vi "Main Tclk.vi"() -> ()   [LabVIEW 2018] (continued)
      n182 = local write "Beam dump at zero"(w117) -> ()
      n183 = local write "EHT off"(w117) -> ()
      n184 = local write "Temperature warning armed"(w117) -> ()
      n185 = local write "Auto Align"(w117) -> ()
      n186 = local write "Auto re-engage"(w117) -> ()
      n187 = local write "Off"(w117) -> ()
      n188 = local write "Spot"(w117) -> ()
      n189 = local write "Auto Stig"(w117) -> ()
      n190 = local write "FIB Profile"(w117) -> ()
      n191 = shared-variable "My Computer\\Zeiss Library.lvlib\\Milling Line Paused"(w117) -> ()  [unwired: 1 in, 1 out]
      n192 = local write "dat to csv and xml"(w117) -> ()
      n193 = local write "Send reheat start email"(w117) -> ()
      n194 = local write "Mouse down"(w117) -> ()
      n195 = call-poly <vilib>:"DAQmx Create Virtual Channel.vi"("physical channels"=w274) -> ("task out"=w272:refnum<k21>, "error out"=w273:errorcluster)  [unwired: 13 in]
      n196 = local write "Mill Stop"(w117) -> ()
      n197 = local write "Stop"(w117) -> ()
      n198 = local write "ROI"(w117) -> ()
      n199 = property on="Reheat Parameters" class="Clust (strict)"("Visible"=w175) -> ()  [unwired: 2 in, 2 out]
      n200 = property on="FIB Parameters" class="Clust (strict)"("Visible"=w177) -> ()  [unwired: 2 in, 2 out]
      n201 = property on="HV Data Output" class="Clust (strict)"("Visible"=w176) -> ()  [unwired: 2 in, 2 out]
      n202 = property on="Capella HV Data Output" class="Clust (strict)"("Visible"=w114) -> ()  [unwired: 2 in, 2 out]
      n203 = Unbundle By Name(w273) -> ("status"=w271:bool)
      n204 = local write "Auto Focus"(w117) -> ()
      n205 = shared-variable "My Computer\\Zeiss Library.lvlib\\Stop"(w117) -> ()  [unwired: 1 in, 1 out]
      n206 = local write "Scan x1"(w117) -> ()
      n207 = local write "FIB time lapse"(w117) -> ()
      n208 = local write "Reheat from last"(w117) -> ()
      n209 = local write "SEM Status"(w326) -> ()
      n210 = local read "FIB Scan Parameters"() -> (w317:T32)
      n211 = expression code="x/2"(w278) -> (w279:dbl)
      n212 = local write "Request to reheat"(w117) -> ()
      n213 = local write "Mill"(w117) -> ()
      n214 = case shown="False" w271 {
        tunnel: w272 -> [w600 _]
        frame False {
          n215 = call <vilib>:"DAQmx Clear Task.vi"("task in"=w600) -> ()  [unwired: 14 in, 1 out]
          n216 = property on="Sweep enabled" class="Bool (strict)"("DisabledEnum"=T44."Enabled" ("Disabled")) -> ()  [unwired: 2 in, 2 out]
        }
        frame True {
          n217 = local write "Sweep enabled"(FALSE ("Sweep enabled")) -> ()
          n218 = property on="Sweep enabled" class="Bool (strict)"("DisabledEnum"=T44."Disabled and Grayed Out" ("Disabled")) -> ()  [unwired: 2 in, 2 out]
        }
      }
      n219 = local write "Re-engage cancelled"(w117) -> ()
      n220 = property on="COM port" class="VISAName"("DisabledEnum"=w277) -> ()  [unwired: 2 in, 2 out]
      n221 = local write "Focus index stop trigger active"(w117) -> ()
      n222 = local read "Milling para"() -> (w313:T35)
      n223 = Bundle By Name(cluster=w313, "FIB FOV (um)"=w278, "Mill from Bottom"=FALSE, "X size (um)"=w279, "Z size (um)"=w279) -> (w312:T35)
      n224 = local read "Alert Settings"() -> (w233:T36)
      n225 = Bundle By Name(cluster=w233, "Low limit"=w232, "High limit"=w231) -> (w230:T36)
      n226 = local read "SEM Options"() -> (w306:T27)
      n227 = property on="Start FIB HV DataLog" class="Bool (strict)"("Visible"=w206) -> ()  [unwired: 2 in, 2 out]
      n228 = property on="Low limit" class="DigNum (strict)"("Caption.Text"=w242) -> ()  [unwired: 2 in, 2 out]
      n229 = property on="High limit" class="DigNum (strict)"("Caption.Text"=w241) -> ()  [unwired: 2 in, 2 out]
      n230 = property on="Faraday Cup (nA)" class="DigNum (strict)"("Caption.Text"=w239) -> ()  [unwired: 2 in, 2 out]
      n231 = property on="Faraday Cup log" class="XYGraph (strict)"("YScale.NameLbl.Text"=w238) -> ()  [unwired: 2 in, 2 out]
      n232 = property on="Config Tabs" class="TabCtl (strict)"() -> ("Pages"=w211:refnum<vi>[])  [unwired: 2 in, 2 out]
      n233 = local write "FIB"(w117) -> ()
      n234 = Bundle By Name(cluster=w317, "X size (V)"=w315, "Z size (V)"=w315) -> (w316:T32)
      n235 = local write "Mill Manual Pause"(w117) -> ()
      n236 = local write "FIB-SEM Angle"(w314) -> ()
      n237 = local read "FIB Options"() -> (w310:T33)
      n238 = property on="SEM HV Data Output" class="Clust (strict)"("Visible"=w114) -> ()  [unwired: 2 in, 2 out]
      n239 = local write "3D FIB-SEM"(w117) -> ()
      n240 = local write "Pause for reheat"(w117) -> ()
      n241 = local write "Request to stop reheat"(w117) -> ()
      n242 = property on="Extractor (kV)" class="DigNum (strict)"("Visible"=w199) -> ()  [unwired: 2 in, 2 out]
      n243 = Bundle By Name(cluster=w310, "Flip x"=w168, "Flip z"=TRUE ("data")) -> (w309:T33)
      n244 = Index Array(array=w211, index=T43."FIB Reheat" ("Config Tabs")) -> (element=w210:refnum<vi>)
      n245 = local write "Alert Settings"(w230) -> ()
      n246 = Bundle By Name(cluster=w306, "Detector A"=w304, "Detector B"=w303) -> (w305:T27)
      n247 = local read "Milling para"() -> (w324:T35)
      n248 = Bundle By Name(cluster=w324, "Auto pause"=w258, "Mill start from Last"=w258) -> (w323:T35)
      n249 = local write "Start Current DataLog"(w117) -> ()
      n250 = xnode "Match Regular Expression"("input string"=w182, "regular expression"="Merlin", "ignore case? (F)"=TRUE) -> ("offset past match"=w269:i32)  [unwired: 3 in, 4 out]
      n251 = xnode "Match Regular Expression"("input string"=w182, "regular expression"="Gemini500", "ignore case? (F)"=TRUE) -> ("offset past match"=w184:i32)  [unwired: 3 in, 4 out]
      n252 = property class="Page"(reference=w210, "PageEnb"=w144) -> ()  [unwired: 1 in, 2 out]
      n253 = local write "FIB Imaging"(w117) -> ()
      n254 = property on="Turn FIB gun standby" class="Bool (strict)"("Visible"=w114) -> ()  [unwired: 2 in, 2 out]
      n255 = local write "FIB Options"(w309) -> ()
      n256 = Equal?(x=w269, y=-1) -> (x = y?=w181:bool)
      n257 = Equal?(x=w184, y=-1) -> (x = y?=w180:bool)
      n258 = local write "FIB Scan Parameters"(w316) -> ()
      n259 = local write "Cancel Auto re-engage"(w117) -> ()
      n260 = property on="13nA Condenser (V)" class="DigNum (strict)"("Visible"=w199) -> ()  [unwired: 2 in, 2 out]
      n261 = local write "Milling para"(w312) -> ()
      n262 = local write "Status message"("standby" ("Status message")) -> ()
      n263 = local write "SEM Options"(w305) -> ()
      n264 = And(x=w181, y=w180) -> (x .and. y?=w179:bool)
      n265 = local write "Reheat completed"(w117) -> ()
      n266 = property on="Status Tabs" class="TabCtl (strict)"() -> ("Pages"=w207:refnum<vi>[])  [unwired: 2 in, 2 out]
      n267 = local write "Unfreeze"(w117) -> ()
      n268 = local write "Scan xn"(w117) -> ()
      n269 = Square Root(x=sgl 2.0 ("t")) -> (sqrt(x)=w118:sgl)
      n270 = local write "Milling para"(w323) -> ()
      n271 = property on="27nA Condenser (V)" class="DigNum (strict)"("Visible"=w199) -> ()  [unwired: 2 in, 2 out]
      n272 = property on="Reheat Output" class="Clust (strict)"("Visible"=w206) -> ()  [unwired: 2 in, 2 out]
      n273 = property on="Turn off FIB gun" class="Bool (strict)"("Visible"=w114) -> ()  [unwired: 2 in, 2 out]
      n274 = property on="Suppressor (V)" class="DigNum (strict)"("Visible"=TRUE) -> ()  [unwired: 2 in, 2 out]
      n275 = Divide(x=w119, y=w118) -> (x/y=w120:sgl)
      n276 = Index Array(array=w207, index=T11."HV Data" ("Status Tabs")) -> (element=w208:refnum<vi>)
      n277 = Select(t=w119, s=w179, f=w120) -> (s? t:f=w178:sgl)
      "X full scale (V)" <- w178
      n278 = property class="DAQmx Device"("Active Device"=w266) -> (error out=w260:errorcluster, "AI.PhysicalChans"=w265:tag[])  [unwired: 2 in, 1 out]
      "Logging Channels" <- w265
      n279 = local read "File Information"() -> (w308:T31)
      n280 = property class="Page"(reference=w208, "PageEnb"=w144) -> ()  [unwired: 1 in, 2 out]
      n281 = shared-variable ".\\Zeiss Library.lvlib\\X full scale (V)"(w178) -> ()  [unwired: 1 in, 1 out]
      n282 = property on="Open FIB gun valve" class="Bool (strict)"("Visible"=w114) -> ()  [unwired: 2 in, 2 out]
      n283 = property on="Image Tabs" class="TabCtl (strict)"() -> ("Pages"=w146:refnum<vi>[])  [unwired: 2 in, 2 out]
      n284 = Unbundle By Name(w260) -> ("status"=w259:bool)
      n285 = Bundle By Name(cluster=w308, "File path"=path "E:/Images", "Save recipe"=w125, "Load recipe"=w125) -> (w307:T31)
      n286 = property on="Cursor Z (V)" class="DigNum (strict)"("Visible"=w125) -> ()  [unwired: 2 in, 2 out]
      n287 = Array Size(array="Parameter Names") -> (size(s)=w262:i32)
      n288 = shared-variable ".\\Zeiss Library.lvlib\\Upload flags path"("D:\\UploadFlags" ("string")) -> ()  [unwired: 1 in, 1 out]
      n289 = property on="FIB Gun Valve Status" class="Str"("Visible"=w114) -> ()  [unwired: 2 in, 2 out]
      n290 = Index Array(array=w146, index=T37."FIB HV Data" ("Image Tabs")) -> (element=w145:refnum<vi>)
      n291 = Array Subset(array=w265, length=w262) -> (w264:tag[])  [unwired: 1 in]
      n292 = Build Path(base path=w129, name or relative path="Email Log") -> (appended path=w215:path)
      "Email Log Files" <- w215
      n293 = Build Path(base path=w129, name or relative path="FIB HV DataLog") -> (appended path=w219:path)
      "FIB HV DataLog Files" <- w219
      n294 = Build Path(base path=w129, name or relative path="SEM HV DataLog") -> (appended path=w169:path)
      "SEM HV DataLog Files" <- w169
      n295 = Build Path(base path=w129, name or relative path="Current DataLog") -> (appended path=w166:path)
      "Current DataLog Files" <- w166
      n296 = Build Path(base path=w129, name or relative path="FIB Reheat Log") -> (appended path=w197:path)
      "FIB Reheat Log Files" <- w197
      n297 = Build Path(base path=w129, name or relative path="Re-engage") -> (appended path=w131:path)
      "Re-engage Files" <- w131
      n298 = Build Path(base path=w129, name or relative path="FIB Probes.csv") -> (appended path=w132:path)
      n299 = Build Path(base path=w129, name or relative path="Last FIB milling snapshot.xml") -> (appended path=→"Last milling snapshot":path)
      n300 = Build Path(base path=w129, name or relative path="Last FIB recipe.csv") -> (appended path=→"Last FIB recipe":path)
      n301 = Build Path(base path=w129, name or relative path="Last FIB image.png") -> (appended path=→"Last FIB image":path)
      n302 = Build Path(base path=w129, name or relative path="Last FIB zoom pre image.png") -> (appended path=→"Last FIB zoom pre image":path)
      n303 = Build Path(base path=w129, name or relative path="Last DetA LM image.png") -> (appended path=→"Last Det A Low Mag":path)
      n304 = Build Path(base path=w129, name or relative path="Last DetB LM image.png") -> (appended path=→"Last Det B Low Mag":path)
      n305 = Build Path(base path=w129, name or relative path="Email alert recipients.txt") -> (appended path=w226:path)
      "Email recipents file" <- w226
      n306 = property class="Page"(reference=w145, "PageEnb"=w144) -> ()  [unwired: 1 in, 2 out]
      n307 = property on="FIB Milling Objective (V)" class="DigNum (strict)"("Visible"=w114) -> ()  [unwired: 2 in, 2 out]
      n308 = property on="FIB Milling Probe" class="CmbBox"("Visible"=w114) -> ()  [unwired: 2 in, 2 out]
      n309 = local write "File Information"(w307) -> ()
      n310 = Path To String(path=w129) -> (string=w130:string)
      n311 = File/Directory Info(path=w215) -> (path out=w212:path, error out=w214:errorcluster)  [unwired: 1 in, 5 out]
      n312 = File/Directory Info(path=w219) -> (path out=w222:path, error out=w220:errorcluster)  [unwired: 1 in, 5 out]
      n313 = File/Directory Info(path=w169) -> (path out=w170:path, error out=w172:errorcluster)  [unwired: 1 in, 5 out]
      n314 = File/Directory Info(path=w166) -> (path out=w165:path, error out=w163:errorcluster)  [unwired: 1 in, 5 out]
      n315 = File/Directory Info(path=w197) -> (path out=w194:path, error out=w196:errorcluster)  [unwired: 1 in, 5 out]
      n316 = File/Directory Info(path=w129) -> (path out=w255:path, error out=w257:errorcluster)  [unwired: 1 in, 5 out]
      n317 = File/Directory Info(path=w131) -> (path out=w236:path, error out=w234:errorcluster)  [unwired: 1 in, 5 out]
      n318 = call-poly <vilib>:"Read From Spreadsheet File.vi"("delimiter (\\t)"="," ("delimiter (\\t)"), "file path (dialog if empty)"=w132) -> ("all rows"=w140:string[][])  [unwired: 5 in, 4 out]
      n319 = call <vilib>:"DAQmx Flatten Channel String.vi"("names in"=w264) -> ("names out"=→"Active logging channels":string)  [unwired: 13 in, 1 out]
      n320 = shared-variable ".\\Zeiss Library.lvlib\\3D FIB-SEM Files Path"(w130) -> ()  [unwired: 1 in, 1 out]
      n321 = File/Directory Info(path=w226) -> (path out=w223:path, error out=w225:errorcluster)  [unwired: 1 in, 5 out]
      n322 = Unbundle By Name(w214) -> ("status"=w213:bool)
      n323 = Unbundle By Name(w220) -> ("status"=w221:bool)
      n324 = Unbundle By Name(w196) -> ("status"=w195:bool)
      n325 = Unbundle By Name(w234) -> ("status"=w235:bool)
      n326 = Array Size(array=w140) -> (size(s)=w138:i32[])
      n327 = Unbundle By Name(w172) -> ("status"=w171:bool)
      n328 = Unbundle By Name(w163) -> ("status"=w164:bool)
      n329 = Unbundle By Name(w257) -> ("status"=w256:bool)
      n330 = property on="Min FIB probe" class="Bool (strict)"("Visible"=w114) -> ()  [unwired: 2 in, 2 out]
      n331 = property on="Save Probe Table" class="Bool (strict)"("Visible"=w114) -> ()  [unwired: 2 in, 2 out]
      n332 = Unbundle By Name(w225) -> ("status"=w224:bool)
      n333 = Index Array(array=w138, index=0) -> (element=w137:i32)
      n334 = Decrement(x=w137) -> (x-1=w141:i32)
      n335 = case shown="True" w213 {
        tunnel: w212 -> [_ w457]
        frame False {
        }
        frame True {
          n336 = Create Folder(path (use dialog)=w457) -> ()  [unwired: 1 in, 4 out]
        }
      }
      n337 = case shown="True" w221 {
        tunnel: w222 -> [_ w458]
        frame False {
        }
        frame True {
          n338 = Create Folder(path (use dialog)=w458) -> ()  [unwired: 1 in, 4 out]
        }
      }
      n339 = case shown="True" w171 {
        tunnel: w170 -> [_ w344]
        frame False {
        }
        frame True {
          n340 = Create Folder(path (use dialog)=w344) -> ()  [unwired: 1 in, 4 out]
        }
      }
      n341 = case shown="True" w164 {
        tunnel: w165 -> [_ w343]
        frame False {
        }
        frame True {
          n342 = Create Folder(path (use dialog)=w343) -> ()  [unwired: 1 in, 4 out]
        }
      }
      n343 = case shown="True" w195 {
        tunnel: w194 -> [_ w456]
        frame False {
        }
        frame True {
          n344 = Create Folder(path (use dialog)=w456) -> ()  [unwired: 1 in, 4 out]
        }
      }
      n345 = case shown="True" w256 {
        tunnel: w255 -> [_ w481]
        frame False {
        }
        frame True {
          n346 = Create Folder(path (use dialog)=w481) -> ()  [unwired: 1 in, 4 out]
        }
      }
      n347 = case shown="True" w235 {
        tunnel: w236 -> [_ w480]
        frame False {
        }
        frame True {
          n348 = Create Folder(path (use dialog)=w480) -> ()  [unwired: 1 in, 4 out]
        }
      }
      n349 = property on="Image Tabs" class="TabCtl (strict)"() -> ("Pages"=w204:refnum<vi>[])  [unwired: 2 in, 2 out]
      n350 = property on="Max FIB probe" class="Bool (strict)"("Visible"=w114) -> ()  [unwired: 2 in, 2 out]
      n351 = Index Array(array=w140, index (row)=w141) -> (element=w135:string[])  [unwired: 1 in]
      n352 = case shown="False" w224 {
        tunnel: w223 -> [w466 _]
        frame False {
          n353 = Open/Create/Replace File(file path (use dialog)=w466) -> (refnum out=w467:refnum<file>, error out=w468:errorcluster)  [unwired: 5 in, 1 out]
          n354 = local read "Mail server"() -> (w463:string)
          n355 = local read "Hardware Configuration"() -> (w461:T25)
          n356 = Read from Text File(file (use dialog)=w467, error in=w468) -> (refnum out=w469:refnum<file>, text=w465:string, error out=w470:errorcluster)  [unwired: 2 in, 1 out]
          n357 = while {
            shift-right: [w478] -> _
            shift-left: w465 -> [w475]
            tunnel: [w477] -> w459 mode=indexing
            stop <- w471 stop-if-true
            n358 = String Length(string=w475) -> (length=w474:i32)
            n359 = Match Pattern(string=w475, regular expression="\n") -> (before substring=w477:string, after substring=w478:string, offset past match=w476:i32)  [unwired: 1 in, 1 out]
            n360 = local read "Off"() -> (w472:bool)
            n361 = Equal?(x=w476, y=w474) -> (x = y?=w473:bool)
            n362 = Or(x=w473, y=w472) -> (x .or. y?=w471:bool)
          }
          n363 = Close File(refnum=w469, error in=w470) -> ()  [unwired: 2 out]
          n364 = Unbundle By Name(w461) -> ("Machine ID"=w462:string)
          n365 = local write "Email Alert Recipients"(w459) -> ()
          n366 = call "Email alert.vi"("Send email"=TRUE, "Machine ID"=w462, "Mail server"=w463, "Alarm message"="3D FIB-SEM restarted", "Recipents"=w459) -> ()  [unwired: 7 in]
        }
        frame True {
        }
      }
      n367 = Delete From Array(array=w135, length=1, index=0) -> (array with subset deleted=w123:string[])  [unwired: 1 out]
      n368 = case shown="False" w259 {
        frame False {
          w482 = TRUE ("Enable logging")
          n369 = local write "Enable logging"(TRUE ("Enable logging")) -> ()
          n370 = property on="Sample rate (Hz)" class="DigNum (strict)"("Visible"=w482) -> ()  [unwired: 2 in, 2 out]
          n371 = property on="Samples size" class="DigNum (strict)"("Visible"=w482) -> ()  [unwired: 2 in, 2 out]
          n372 = property on="Logging Channels" class="Arr (strict)"("Visible"=w482) -> ()  [unwired: 2 in, 2 out]
          n373 = property on="Parameter Names" class="Arr (strict)"("Visible"=w482) -> ()  [unwired: 2 in, 2 out]
          n374 = property on="Measurements" class="WFChart (strict)"("Visible"=w482) -> ()  [unwired: 2 in, 2 out]
          n375 = property on="Clear" class="Bool"("Visible"=w482) -> ()  [unwired: 2 in, 2 out]
          n376 = property on="Enable logging" class="Bool (strict)"("DisabledEnum"=T44."Enabled" ("Disabled")) -> ()  [unwired: 2 in, 2 out]
        }
        frame True {
          w485 = FALSE ("Enable logging")
          n377 = local write "Enable logging"(FALSE ("Enable logging")) -> ()
          n378 = property on="Sample rate (Hz)" class="DigNum (strict)"("Visible"=w485) -> ()  [unwired: 2 in, 2 out]
          n379 = property on="Samples size" class="DigNum (strict)"("Visible"=w485) -> ()  [unwired: 2 in, 2 out]
          n380 = property on="Logging Channels" class="Arr (strict)"("Visible"=w485) -> ()  [unwired: 2 in, 2 out]
          n381 = property on="Parameter Names" class="Arr (strict)"("Visible"=w485) -> ()  [unwired: 2 in, 2 out]
          n382 = property on="Measurements" class="WFChart (strict)"("Visible"=w485) -> ()  [unwired: 2 in, 2 out]
          n383 = property on="Clear" class="Bool"("Visible"=w485) -> ()  [unwired: 2 in, 2 out]
          n384 = property on="Enable logging" class="Bool (strict)"("DisabledEnum"=T44."Disabled and Grayed Out" ("Disabled")) -> ()  [unwired: 2 in, 2 out]
        }
      }
      n385 = property on="FIB probe switching" class="Str"("Visible"=w114) -> ()  [unwired: 2 in, 2 out]
      n386 = Index Array(array=w204, index=T37."FIB Milling Offset after Pause" ("Image Tabs")) -> (element=w203:refnum<vi>)
      n387 = Build Cluster Array(w123, w123) -> (w122:cluster{"String":string, "String":string}[])
      n388 = property class="Page"(reference=w203, "PageVis"=FALSE ("Page Visible")) -> ()  [unwired: 1 in, 2 out]
      n389 = local read "FIB Scan Parameters"() -> (w152:T32)
      n390 = property on="FIB Milling Probe" class="CmbBox"("Strings And Values[]"=w122) -> ()  [unwired: 2 in, 2 out]
      n391 = shared-variable "My Computer\\Zeiss Library.lvlib\\FIB Probes"(w123) -> ()  [unwired: 1 in, 1 out]
      n392 = local read "Milling para"() -> (w160:T35)
      n393 = control-ref of="FIB Image"() -> (w161:refnum<vi>)
      n394 = local read "FIB Scan Parameters"() -> (w159:T32)
      n395 = local read "FIB Options"() -> (w158:T33)
      n396 = shared-variable ".\\Zeiss Library.lvlib\\Milling Z Voltage RT"() -> (w156:sgl)  [unwired: 1 in, 1 out]
      n397 = property on="FIB HV target matched" class="Bool (strict)"("Visible"=w114) -> ()  [unwired: 2 in, 2 out]
      n398 = property on="Get V/I slope" class="Bool (strict)"("Visible"=w114) -> ()  [unwired: 2 in, 2 out]
      n399 = Unbundle By Name(w152) -> ("Z resolution"=w151:u32, "X resolution"=w150:u32)
      n400 = property on="FIB probe auto min" class="Bool (strict)"("Visible"=w114) -> ()  [unwired: 2 in, 2 out]
      n401 = property on="FIB V/I slope" class="DigNum (strict)"("Visible"=w114) -> ()  [unwired: 2 in, 2 out]
      n402 = call "FIB image draw milling.vi"("Milling Z Voltage"=w156, "Milling para"=w160, "FIB Options"=w158, "FIB Scan Parameters"=w159, "Origin"=TRUE, "Image reference"=w161) -> ("Trapezoidal"=w155:cluster{"X":i16, "Y":i16}[])  [unwired: 4 in, 1 out]
      n403 = Initialize Array(i16 0 ("element"), w151, w150) -> (w154:i16[][])
      n404 = local write "Trapezoidal"(w155) -> ()
      n405 = local write "FIB Image"(w154) -> ()
      n406 = property on="Mill start from Last" class="Bool (strict)"("DisabledEnum"=w116) -> ()  [unwired: 2 in, 2 out]
      n407 = property on="Scan x1" class="Bool (strict)"("DisabledEnum"=w116) -> ()  [unwired: 2 in, 2 out]
      n408 = property on="Scan xn" class="Bool (strict)"("DisabledEnum"=w116) -> ()  [unwired: 2 in, 2 out]
      n409 = property on="FIB Imaging" class="Bool (strict)"("DisabledEnum"=w116) -> ()  [unwired: 2 in, 2 out]
      n410 = property on="FIB time lapse" class="Bool (strict)"("DisabledEnum"=w116) -> ()  [unwired: 2 in, 2 out]
      n411 = property on="Reset" class="Bool (strict)"("DisabledEnum"=w116) -> ()  [unwired: 2 in, 2 out]
      n412 = property on="Pre image" class="Bool (strict)"("DisabledEnum"=w116) -> ()  [unwired: 2 in, 2 out]
      n413 = property on="Post image" class="Bool (strict)"("DisabledEnum"=w116) -> ()  [unwired: 2 in, 2 out]
      n414 = property on="Mill" class="Bool (strict)"("DisabledEnum"=w116) -> ()  [unwired: 2 in, 2 out]
      n415 = property on="Mill Manual Pause" class="Bool (strict)"("DisabledEnum"=w116) -> ()  [unwired: 2 in, 2 out]
      n416 = property on="Z-step (nm)" class="DigNum (strict)"("DisabledEnum"=w116) -> ()  [unwired: 2 in, 2 out]
      n417 = property on="X min index" class="DigNum (strict)"("Visible"=w240) -> ()  [unwired: 2 in, 2 out]
      n418 = property on="X max index" class="DigNum (strict)"("Visible"=w240) -> ()  [unwired: 2 in, 2 out]
      n419 = property on="AF Steps" class="DigNum (strict)"("DisabledEnum"=w116) -> ()  [unwired: 2 in, 2 out]
      n420 = property on="AS Steps" class="DigNum (strict)"("DisabledEnum"=w116) -> ()  [unwired: 2 in, 2 out]
      n421 = property on="AA Steps" class="DigNum (strict)"("DisabledEnum"=w116) -> ()  [unwired: 2 in, 2 out]
      n422 = property on="Start Current DataLog" class="Bool (strict)"("DisabledEnum"=w116) -> ()  [unwired: 2 in, 2 out]
      n423 = property on="Detector C name" class="Str"("DisabledEnum"=w217) -> ()  [unwired: 2 in, 2 out]
      n424 = property on="Detector D name" class="Str"("DisabledEnum"=w217) -> ()  [unwired: 2 in, 2 out]
      n425 = property on="Pause for reheat" class="Bool (strict)"("DisabledEnum"=w217) -> ()  [unwired: 2 in, 2 out]
      n426 = property on="Request to stop reheat" class="Bool (strict)"("DisabledEnum"=w217) -> ()  [unwired: 2 in, 2 out]
      "3D FIB-SEM Files" <- w129
      "Reheat complete file" <- path "C:/Program Files (x86)/FEI Company/BDS/Reheat/Complete.txt" ("Log file path")
      "Reheat stopped file" <- path "C:/Program Files (x86)/FEI Company/BDS/Reheat/Stopped.txt" ("Log file path")
      "FIB emission below limit counts" <- w113
      "FI below limit counts" <- w113
      "WD array tiled" <- w189
      "ASX Success tiled" <- w193
      "ASY Success tiled" <- w193
      "AAX Success tiled" <- w193
      "AAY Success tiled" <- w193
      "AF Success tiled" <- w193
      "FI array" <- w127
      "FI grid array" <- w189
      "FI array tiled" <- w189
      "FI grid array tiled" <- sgl[][][][][] [] ("FI grid array tiled")
      "Best WD FI tiled" <- w191
      "Best WD (mm) tiled" <- w191
      "Slope tiled" <- w191
      "StigX array tiled" <- w189
      "Best Stig X FI tiled" <- w191
      "Best Stig X (%) tiled" <- w191
      "StigY array tiled" <- w189
      "AlnX array tiled" <- w189
      "AlnY array tiled" <- w189
      "Best Stig Y FI tiled" <- w191
      "Best Stig Y (%) tiled" <- w191
      "Best Aln X FI tiled" <- w191
      "Best Aln X (%) tiled" <- w191
      "Best Aln Y FI tiled" <- w191
      "Best Aln Y (%) tiled" <- w191
      "Skip Steps tiled" <- u8[][] [] ("FI array")
      "FIB CL I out of bound counts" <- w113
      "AF Count" <- w113
      "AS Count" <- w113
      "AA Count" <- w113
      "WD Stig Aln tile offsets" <- T42 {[], [], [], [], [], [], []} ("output cluster")
      "Reheat start file" <- path "C:/Program Files (x86)/FEI Company/BDS/Reheat/Start.txt" ("Log file path")
      "Milling mode" <- T10."FIB" ("FIB mode")
      "LM overhead" <- w113
      "MM overhead" <- w113
      "Re-engage counts" <- w113
      "Recovered counts" <- w113
      "Last re-engage count" <- w113
      "FIB slice #" <- w113
      "3D image paused active" <- w117
      "FIB probe switching" <- "Go to                 or               current of the same probe " ("FIB probe switching")
      "FIB suppressor below limit counts" <- w113
      "Continued fine milling frames" <- w113
    }
    frame #2 {
      n427 = flat-sequence {
        frame #0 {
          n428 = local read "Post #1up"() -> (w694:tag)
          n429 = local read "Post #1down"() -> (w695:tag)
          n430 = local read "Post #2up"() -> (w696:tag)
          n431 = local read "Post #2down"() -> (w697:tag)
          n432 = call "SEM shutter.vi"("Shutter close"=TRUE, "Shutter AO4"=w697, "Shutter AO3"=w696, "Shutter AO2"=w695, "Shutter AO1"=w694) -> ()  [unwired: 6 in, 1 out]
        }
        frame #1 {
          w698 = 10.0 ("Output voltage (V)")
          n433 = local read "Hardware Configuration"() -> (w701:T25)
          n434 = Unbundle By Name(w701) -> ("SEM X coil"=w700:refnum<k15>, "SEM Y coil"=w699:refnum<k15>)
          n435 = call "FGEN DC voltage.vi"("Output voltage (V)"=w698, "Resource Name"=w700) -> ()  [unwired: 9 in, 1 out]
          n436 = call "FGEN DC voltage.vi"("Output voltage (V)"=w698, "Resource Name"=w699) -> ()  [unwired: 9 in, 1 out]
        }
        frame #2 {
          n437 = local read "Post #1up"() -> (w703:tag)
          n438 = local read "Post #1down"() -> (w704:tag)
          n439 = local read "Post #2up"() -> (w705:tag)
          n440 = local read "Post #2down"() -> (w706:tag)
          n441 = call "SEM shutter.vi"("Shutter close"=FALSE, "Shutter AO4"=w706, "Shutter AO3"=w705, "Shutter AO2"=w704, "Shutter AO1"=w703) -> ()  [unwired: 6 in, 1 out]
        }
      }
    }
    frame #3 {
      w708 = u32 0 ("FIB slice #")
      n442 = Current VI's Path() -> (path=w710:path)
      n443 = while {
        shift-right: [w2611] -> _
        shift-left: _ -> [w2610]
        shift-right: [w2586] -> _
        shift-left: _ -> [w2587]
        shift-right: [w2580] -> _
        shift-left: _ -> [w2579]
        shift-right: [w2569] -> _
        shift-left: _ -> [w2572]
        stop <- "Stop" stop-if-true
        w2493 = sgl 5.0 ("y")
        w2498 = sgl 5.0 ("y")
        n444 = local read "SEM Status"() -> (w2603:T12)
        n445 = shared-variable ".\\Zeiss Library.lvlib\\SEMInfo"() -> (w2611:variant)  [unwired: 2 out]
        n446 = shared-variable ".\\Zeiss Library.lvlib\\Det A Img"() -> (w2586:i16[][])  [unwired: 2 out]
        n447 = shared-variable ".\\Zeiss Library.lvlib\\Det B Img"() -> (w2580:i16[][])  [unwired: 2 out]
        n448 = shared-variable ".\\Zeiss Library.lvlib\\FIB Img"() -> (w2569:i16[][])  [unwired: 1 in, 1 out]
        n449 = local read "SEM Scan Parameters"() -> (w2618:T26)
        n450 = local read "Hardware Configuration"() -> (w2505:T25)
        n451 = local read "SEM Scan Parameters"() -> (w2521:T26)
        n452 = local read "SEM Options"() -> (w2504:T27)
        n453 = local read "SEM Status"() -> (w2503:T12)
        n454 = local read "X full scale (V)"() -> (w2502:sgl)
        n455 = local read "Mid Mag SEM"() -> (w2506:T29)
        n456 = local read "SEM Mid Mag Scan Parameters"() -> (w2507:T5)
        n457 = shared-variable ".\\Zeiss Library.lvlib\\Tiled Image fit to"("Tiled Image fit to") -> ()  [unwired: 1 in, 1 out]
        n458 = Wait Until Next ms Multiple(millisecond multiple=u32 100) -> ()  [unwired: 1 out]
        n459 = Variant To Data(type=w2603, Variant=w2611) -> (data=w2602:T12)  [unwired: 1 in, 1 out]
        n460 = Equal?(x=w2611, y=w2610) -> (x = y?=w2606:bool)
        n461 = local read "Status message"() -> (w2460:string)
        n462 = Unbundle By Name(w2506) -> ("X size (um)"=w2510:sgl, "Y size (um)"=w2511:sgl, "X center (um)"=w2512:dbl, "Y center (um)"=w2513:dbl, "Mid mag scan rate (Hz)"=w2508:u32, "Pixel size (nm)"=w2509:sgl)
        n463 = Equal?(x=w2587, y=w2586) -> (x = y?=w2585:bool[][])
        n464 = Equal?(x=w2579, y=w2580) -> (x = y?=w2584:bool[][])
        n465 = Equal?(x=w2572, y=w2569) -> (x = y?=w2571:bool[][])
        n466 = Unbundle By Name(w2618) -> ("Scan rate (Hz)"=w2622:u32, "X size (um)"=w2485:sgl, "Y size (um)"=w2482:sgl, "Frame line rampdown ratio"=w2623:sgl, "Pixel size (nm)"=w2486:sgl)
        n467 = And Array Elements(Boolean array=w2585) -> (logical AND=w2583:bool)
        n468 = And Array Elements(Boolean array=w2584) -> (logical AND=w2582:bool)
        n469 = And Array Elements(Boolean array=w2571) -> (logical AND=w2570:bool)
        n470 = Unbundle By Name(w2602) -> ("Remaining time (m)"=w2609:u16, "Remaining time (s)"=w2608:u8)
        n471 = call "SEM Scan Parameter Coerce.vi"("X full scale (V)"=w2502, "AI upper limit"=50000000.0, "SEM Status"=w2503, "SEM Options"=w2504, "SEM Scan Parameters"=w2521, "Hardware Configuration"=w2505) -> ("Coerced SEM Scan Parameters"=w2469:T5, "SEM FOV"=→"SEM FOV":dbl, "Detector number"=w2522:i16)  [unwired: 3 in]
        n472 = And(x=w2583, y=w2582) -> (x .and. y?=w2581:bool)
        n473 = Unbundle By Name("FIB Options") -> ("Det"=w2597:u16)
        n474 = expression code="x/1000"(w2486) -> (w2481:sgl)
        n475 = case shown="False" w2581 {
          tunnel: w2586 -> [w2870 _]
          tunnel: w2580 -> [w2869 _]
          tunnel: w2460 -> [w2868 _]
          frame False {
            n476 = case shown="\"SEM Low Mag Scan\"" w2868 {
              tunnel: w2869 -> [w2872 w2873]
              tunnel: w2870 -> [w2871 w2874]
              frame Default {
                "Detector B" <- w2872
                "Detector A" <- w2871
              }
              frame "SEM Low Mag Scan" {
                "Detector A Low Mag" <- w2874
                "Det A LM" <- w2874
                "Detector B Low Mag" <- w2873
                "Det B LM" <- w2873
              }
            }
          }
          frame True {
            n477 = shared-variable "My Computer\\Zeiss Library.lvlib\\DetA-scaling"() -> (→"DetA e- Scaling":sgl)  [unwired: 1 in, 1 out]
            n478 = shared-variable "My Computer\\Zeiss Library.lvlib\\DetB-Scaling"() -> (→"DetB e- Scaling":sgl)  [unwired: 1 in, 1 out]
          }
        }
        n479 = case shown="False" w2570 {
          tunnel: w2569 -> [w2855 _]
          frame False {
            n480 = Build Array("Pre image", "Post image") -> (w2857:bool[])
            n481 = Boolean Array To Number(Boolean array=w2857) -> (number=w2856:u32)
            n482 = case shown="0, Default" w2856 {
              tunnel: w2855 -> [w2860 w2861 w2862]
              frame 0, Default {
                "FIB Image" <- w2860
              }
              frame 1 {
                "Pre Image" <- w2861
              }
              frame 2 {
                "Post Image" <- w2862
              }
            }
          }
          frame True {
          }
        }
        n483 = Bundle By Name(cluster=w2507, "X size (um)"=w2510, "Y size (um)"=w2511, "X center (um)"=w2512, "Y center (um)"=w2513, "Scan rate (Hz)"=w2508, "Pixel size (nm)"=w2509, "X size auto"=TRUE) -> (w2514:T5)
        n484 = shared-variable ".\\Zeiss Library.lvlib\\Det"(w2597) -> ()  [unwired: 1 in, 1 out]
        n485 = Add(x=w2609, y=w2608) -> (x+y=w2607:u16)
        n486 = Equal To 0?(x=w2607) -> (x = 0?=w2605:bool)
        n487 = Divide(x=w2485, y=w2481) -> (x/y=w2484:sgl)
        n488 = Increment(x=w2623) -> (x+1=w2619:sgl)
        n489 = Divide(x=w2482, y=w2481) -> (x/y=w2483:sgl)
        n490 = To Double Precision Float(number=w2622) -> (double precision float=w2621:dbl)
        n491 = Reciprocal(x=w2621) -> (1/x=w2620:dbl)
        n492 = Multiply(x=w2484, y=w2619) -> (x*y=w2616:sgl)
        n493 = Multiply(x=w2484, y=w2483) -> (x*y=w2617:sgl)
        n494 = And(x=w2606, y=w2605) -> (x .and. y?=w2604:bool)
        n495 = call "SEM Scan Parameter Coerce.vi"("X full scale (V)"=w2502, "SEM Status"=w2503, "SEM Options"=w2504, "SEM Scan Parameters"=w2514, "Hardware Configuration"=w2505) -> ("Coerced SEM Scan Parameters"=w2468:T5)  [unwired: 4 in, 2 out]
        n496 = Unbundle By Name(w2468) -> ("X size (um)"=w2515:sgl, "Y size (um)"=w2516:sgl, "X center (um)"=w2517:dbl, "Y center (um)"=w2518:dbl, "Scan rate (Hz)"=w2519:u32, "Pixel size (nm)"=w2520:sgl)
        n497 = Bundle By Name(cluster=w2506, "X size (um)"=w2515, "Y size (um)"=w2516, "X center (um)"=w2517, "Y center (um)"=w2518, "Mid mag scan rate (Hz)"=w2519, "Pixel size (nm)"=w2520) -> (w2467:T29)
        n498 = Compound Arithmetic op=MULTIPLY(w2620, w2616, w2483) -> (w2625:dbl)
        "SEM scan time" <- w2625
        n499 = local read "Alert Settings"() -> (w2464:T36)
        n500 = Quotient & Remainder(x=w2625, y=60.0) -> (x-y*floor(x/y)=w2627:dbl, floor(x/y)=w2628:dbl)
        n501 = To Variant(anything="FIB Scan Parameters") -> (Variant=w2598:variant)
        n502 = local read "SEM Status"() -> (w2626:T12)
        n503 = case shown="Default" w2460 {
          frame "SEM Low Mag Scan" {
          }
          frame Default {
            n504 = shared-variable ".\\Zeiss Library.lvlib\\Det A Img Tiled"() -> (→"Det A":i16[][])  [unwired: 1 in, 1 out]
            n505 = shared-variable ".\\Zeiss Library.lvlib\\Det B Img Tiled"() -> (→"Det B":i16[][])  [unwired: 1 in, 1 out]
          }
        }
        n506 = Bundle By Name(cluster=w2626, "Scan time (s)"=w2627, "Scan time (m)"=w2628, "Detector #"=w2522) -> (w2613:T12)
        n507 = property on="Total pixels recorded" class="Slide (strict)"("Scale.Maximum"=w2617) -> ()  [unwired: 2 in, 2 out]
        n508 = local read "Load recipe"() -> (w2531:bool)
        n509 = Unbundle By Name(w2464) -> ("Focus index low limit"=w2465:sgl, "Focus index stop limit"=w2466:sgl)
        n510 = shared-variable ".\\Zeiss Library.lvlib\\Realtime Imaging Scan Para"(w2598) -> ()  [unwired: 1 in, 1 out]
        n511 = To Variant(anything=w2613) -> (Variant=w2612:variant)
        n512 = case shown="True" w2604 {
          tunnel: w2613 -> [_ w2919]
          tunnel: w2612 -> [_ w2918]
          tunnel: w2602 -> [w2917 _]
          frame False {
            "SEM Status" <- w2917
          }
          frame True {
            n513 = shared-variable ".\\Zeiss Library.lvlib\\SEMInfo"(w2918) -> ()  [unwired: 2 out]
            n514 = local write "SEM Status"(w2919) -> ()
          }
        }
        n515 = local read "Low Mag SEM"() -> (w2430:T30)
        n516 = local read "SEM Low Mag Scan Parameters"() -> (w2429:T5)
        n517 = local read "SEM Mid Mag Scan Parameters"() -> (w2428:T5)
        n518 = In Range and Coerce(upper limit=w2465, x=w2466, lower limit=sgl 0.0) -> (coerced(x)=w2463:sgl)  [unwired: 1 out]
        n519 = Bundle By Name(cluster=w2464, "Focus index stop limit"=w2463) -> (w2462:T36)
        n520 = Unbundle By Name(w2430) -> ("Low mag scan"=w2548:bool, "Show HM box"=w2568:bool)
        n521 = property on="Sweep direction" class="Bool (strict)"("Visible"="Sweep enabled") -> ()  [unwired: 2 in, 2 out]
        n522 = property on="Sweep rate (Hz)" class="DigNum (strict)"("Visible"="Sweep enabled") -> ()  [unwired: 2 in, 2 out]
        n523 = property on="Level #" class="DigNum (strict)"("Visible"="Sweep enabled") -> ()  [unwired: 2 in, 2 out]
        n524 = property on="Sweep #" class="DigNum (strict)"("Visible"="Sweep enabled") -> ()  [unwired: 2 in, 2 out]
        n525 = local read "Milling para"() -> (w2533:T35)
        n526 = case shown="False" w2531 {
          tunnel: w2533 -> [w2757 _]
          tunnel: w2469 -> [w2755 _]
          tunnel: w2468 -> [w2754 _]
          tunnel: w2467 -> [w2753 _]
          tunnel: w2462 -> [w2751 _]
          frame False {
            n527 = local write "SEM Scan Parameters"(w2755) -> ()
            n528 = local write "SEM Mid Mag Scan Parameters"(w2754) -> ()
            n529 = local write "Mid Mag SEM"(w2753) -> ()
            n530 = shared-variable ".\\Zeiss Library.lvlib\\FIB PID reset"() -> (w2752:bool)  [unwired: 1 in, 1 out]
            n531 = Bundle By Name(cluster=w2757, "FIB PID reset"=w2752) -> (w2756:T35)
            n532 = local write "Alert Settings"(w2751) -> ()
            n533 = local write "Milling para"(w2756) -> ()
          }
          frame True {
          }
        }
        n534 = Unbundle By Name(w2429) -> ("Scan rate (Hz)"=w2431:u32, "X size (um)"=w2435:sgl, "Y size (um)"=w2439:sgl, "Pixel size (nm)"=w2434:sgl)
        n535 = Unbundle By Name(w2428) -> ("Scan rate (Hz)"=w2536:u32, "X size (um)"=w2479:sgl, "Y size (um)"=w2475:sgl, "Pixel size (nm)"=w2480:sgl)
        n536 = case shown="False" w2548 {
          tunnel: [T44."Disabled and Grayed Out" ("Disabled") T44."Enabled" ("Disabled")] -> w2567
          tunnel: w2430 -> [w2865 _]
          frame False {
            n537 = Bundle By Name(cluster=w2865, "Show HM box"=FALSE) -> (w2863:T30)
            n538 = local write "Low Mag SEM"(w2863) -> ()
          }
          frame True {
          }
        }
        n539 = property on="Focus (V)" class="DigNum (strict)"("Visible"="Sweep enabled") -> ()  [unwired: 2 in, 2 out]
        n540 = property on="Angle (V)" class="DigNum (strict)"("Visible"="Sweep enabled") -> ()  [unwired: 2 in, 2 out]
        n541 = property on="Position (V)" class="DigNum (strict)"("Visible"="Sweep enabled") -> ()  [unwired: 2 in, 2 out]
        n542 = property on="Imbalance (V)" class="DigNum (strict)"("Visible"="Sweep enabled") -> ()  [unwired: 2 in, 2 out]
        n543 = Unbundle By Name(w2533) -> ("X offset (um)"=w2575:sgl, "Z offset (um)"=w2576:sgl, "FIB FOV (um)"=w2441:sgl, "Line milling time (s)"=w2589:sgl, "Lines auto pause"=w2565:u16, "FIB PID on"=w2563:bool, "FIB PID measured"=w2489:u8, "FIB PID target"=w2562:sgl, "FIB PID target slope"=w2532:sgl, "FIB PID P"=w2561:sgl, "FIB PID I"=w2560:sgl, "FIB PID D"=w2559:sgl)  [unwired: 1 out]
        "Lines auto pause" <- w2565
        n544 = expression code="x/1000"(w2434) -> (w2438:sgl)
        n545 = expression code="x/1000"(w2480) -> (w2476:sgl)
        n546 = expression code="x*4735.8+30400"("Extractor (kV)") -> (w2499:sgl)
        n547 = expression code="x*4735.8+30420"("Extractor (kV)") -> (w2492:sgl)
        n548 = To Double Precision Float(number=w2431) -> (double precision float=w2432:dbl)
        n549 = To Double Precision Float(number=w2536) -> (double precision float=w2535:dbl)
        n550 = Divide(x=w2435, y=w2438) -> (x/y=w2436:sgl)
        n551 = Divide(x=w2479, y=w2476) -> (x/y=w2478:sgl)
        n552 = Reciprocal(x=w2432) -> (1/x=w2433:dbl)
        n553 = Divide(x=w2439, y=w2438) -> (x/y=w2437:sgl)
        n554 = Reciprocal(x=w2535) -> (1/x=w2534:dbl)
        n555 = Divide(x=w2475, y=w2476) -> (x/y=w2477:sgl)
        n556 = Divide(x=w2575, y=w2441) -> (x/y=w2577:sgl)
        n557 = Divide(x=w2576, y=w2441) -> (x/y=w2578:sgl)
        n558 = Compound Arithmetic op=MULTIPLY(w2433, w2436, w2437) -> (→"LM SEM scan time":dbl)
        n559 = Compound Arithmetic op=MULTIPLY(w2534, w2478, w2477) -> (→"MM SEM scan time":dbl)
        n560 = Divide(x=w2499, y=w2498) -> (x/y=w2497:sgl)
        n561 = Divide(x=w2492, y=w2493) -> (x/y=w2494:sgl)
        n562 = expression code="x*2"(w2577) -> (w2574:sgl)
        n563 = expression code="x*2"(w2578) -> (w2573:sgl)
        n564 = Round To Nearest(number=w2497) -> (nearest integer value=w2496:sgl)
        n565 = Round To Nearest(number=w2494) -> (nearest integer value=w2495:sgl)
        n566 = shared-variable ".\\Zeiss Library.lvlib\\FIB PID on"(w2563) -> ()  [unwired: 1 in, 1 out]
        n567 = shared-variable "My Computer\\Zeiss Library.lvlib\\FIB PID measured"(w2489) -> ()  [unwired: 1 in, 1 out]
        n568 = shared-variable "My Computer\\Zeiss Library.lvlib\\FIB PID target"(w2562) -> ()  [unwired: 1 in, 1 out]
        n569 = shared-variable "My Computer\\Zeiss Library.lvlib\\FIB PID target slope"(w2532) -> ()  [unwired: 1 in, 1 out]
        n570 = shared-variable "My Computer\\Zeiss Library.lvlib\\FIB PID-I"(w2560) -> ()  [unwired: 1 in, 1 out]
        n571 = shared-variable "My Computer\\Zeiss Library.lvlib\\FIB PID-D"(w2559) -> ()  [unwired: 1 in, 1 out]
        n572 = shared-variable "My Computer\\Zeiss Library.lvlib\\FIB PID-P"(w2561) -> ()  [unwired: 1 in, 1 out]
        n573 = Multiply(x=w2496, y=w2498) -> (x*y=→"13nA Condenser (V)":sgl)
        n574 = Multiply(x=w2495, y=w2493) -> (x*y=→"27nA Condenser (V)":sgl)
        n575 = property on="Show HM box" class="Bool (strict)"("DisabledEnum"=w2567) -> ()  [unwired: 2 in, 2 out]
        n576 = shared-variable ".\\Zeiss Library.lvlib\\Milling X Offset"(w2574) -> ()  [unwired: 1 in, 1 out]
        n577 = shared-variable "My Computer\\Zeiss Library.lvlib\\Milling Z Offset"(w2573) -> ()  [unwired: 1 in, 1 out]
        n578 = shared-variable "My Computer\\Zeiss Library.lvlib\\Line Milling Time (s)"(w2589) -> ()  [unwired: 1 in, 1 out]
        n579 = shared-variable "My Computer\\Zeiss Library.lvlib\\Milling Lines Auto Pause"(w2565) -> ()  [unwired: 1 in, 1 out]
        n580 = shared-variable "My Computer\\Zeiss Library.lvlib\\FIB FOV (um)"(w2441) -> ()  [unwired: 1 in, 1 out]
        n581 = case shown="True" w2568 {
          tunnel: [w2877 w2883] -> w2553
          tunnel: [w2877 w2882] -> w2554
          frame False {
            n582 = call <vilib>:"Draw Rectangle.vi"("picture"=picture data[5B], "rect"=T46 {"left"=0, "top"=0, "right"=0, "bottom"=0}) -> ("new picture"=w2877:picture)  [unwired: 7 in]
          }
          frame True {
            w2895 = T46 {"left"=0, "top"=0, "right"=0, "bottom"=0} ("rect")
            n583 = property on="Det A LM" class="IntGraph (strict)"() -> ("Width"=w2909:u32, "Height"=w2913:u32)  [unwired: 2 in, 2 out]
            n584 = local read "Low Mag SEM"() -> (w2885:T30)
            n585 = local read "SEM Scan Parameters"() -> (w2910:T26)
            n586 = property on="Detector A Low Mag" class="IntGraph (strict)"() -> ("Width"=w2889:u32, "Height"=w2888:u32)  [unwired: 2 in, 2 out]
            n587 = Unbundle By Name(w2885) -> ("Low mag scan FOV (micron)"=w2884:dbl)
            n588 = Unbundle By Name(w2910) -> ("X center (um)"=w2914:sgl, "Y center (um)"=w2915:sgl, "X size (um)"=w2881:sgl, "Y size (um)"=w2880:sgl)
            n589 = expression code="x/2"(w2884) -> (w2916:dbl)
            n590 = Divide(x=w2914, y=w2916) -> (x/y=w2891:dbl)
            n591 = Divide(x=w2915, y=w2916) -> (x/y=w2887:dbl)
            n592 = Divide(x=w2881, y=w2916) -> (x/y=w2890:dbl)
            n593 = Divide(x=w2880, y=w2916) -> (x/y=w2886:dbl)
            n594 = call "CenterSize to StartEnd or Rect-4C.vi"("Resolution"=w2909, "Size"=w2890, "Center"=w2891) -> ("Rect-4C"=w2912:cluster{"left":i16, "right":i16})  [unwired: 2 in, 2 out]
            n595 = call "CenterSize to StartEnd or Rect-4C.vi"("Resolution"=w2913, "Size"=w2886, "Center"=w2887) -> ("Rect-4C"=w2911:cluster{"left":i16, "right":i16})  [unwired: 2 in, 2 out]
            n596 = call "CenterSize to StartEnd or Rect-4C.vi"("Resolution"=w2889, "Size"=w2890, "Center"=w2891) -> ("Rect-4C"=w2896:cluster{"left":i16, "right":i16})  [unwired: 2 in, 2 out]
            n597 = call "CenterSize to StartEnd or Rect-4C.vi"("Resolution"=w2888, "Size"=w2886, "Center"=w2887) -> ("Rect-4C"=w2897:cluster{"left":i16, "right":i16})  [unwired: 2 in, 2 out]
            n598 = Unbundle(w2912) -> ("left"=w2906:i16, "right"=w2905:i16)
            n599 = Unbundle(w2911) -> ("left"=w2904:i16, "right"=w2903:i16)
            n600 = Unbundle(w2896) -> ("left"=w2898:i16, "right"=w2899:i16)
            n601 = Unbundle(w2897) -> ("left"=w2900:i16, "right"=w2901:i16)
            n602 = Bundle By Name(cluster=w2895, "left"=w2906, "right"=w2905, "top"=w2904, "bottom"=w2903) -> (w2902:T46)
            n603 = Bundle By Name(cluster=w2895, "left"=w2898, "right"=w2899, "top"=w2900, "bottom"=w2901) -> (w2892:T46)
            n604 = call <vilib>:"Draw Rectangle.vi"("picture"=picture data[5B], "rect"=w2902, "color(black)"=u32 16776960) -> ("new picture"=w2882:picture)  [unwired: 6 in]
            n605 = call <vilib>:"Draw Rectangle.vi"("picture"=picture data[5B], "rect"=w2892, "color(black)"=u32 16776960) -> ("new picture"=w2883:picture)  [unwired: 6 in]
          }
        }
        n606 = local read "Focus Index Options"() -> (w2402:T28)
        n607 = shared-variable ".\\Zeiss Library.lvlib\\Focus Index Array"() -> (w2458:variant)  [unwired: 1 in, 1 out]
        n608 = shared-variable ".\\Zeiss Library.lvlib\\FIB PID feedback"() -> (→"PID feedback (V)":dbl)  [unwired: 1 in, 1 out]
        n609 = shared-variable "My Computer\\Zeiss Library.lvlib\\FIB PID feedback mean"() -> (→"PID feedback mean (V)":dbl)  [unwired: 1 in, 1 out]
        n610 = local read "Alert Settings"() -> (w2530:T36)
        n611 = shared-variable "My Computer\\Zeiss Library.lvlib\\Focus Index Detector"("FI Detector") -> ()  [unwired: 1 in, 1 out]
        n612 = Unbundle By Name(w2402) -> ("Show Focus Index"=w2401:bool)
        n613 = Variant To Data(type="Image Focus Index Array", Variant=w2458) -> (data=w2457:T15, error out=w2453:errorcluster)  [unwired: 1 in]
        n614 = Unbundle By Name(w2530) -> ("Focus index low limit"=w2529:sgl)
        n615 = shared-variable ".\\Zeiss Library.lvlib\\Focus Index Array"() -> ()  [unwired: 1 in, 2 out]
        n616 = call <vilib>:"Clear Errors.vi"("error in (no error)"=w2453) -> ()  [unwired: 5 in, 2 out]
        n617 = Unbundle By Name(w2453) -> ("status"=w2455:bool)
        n618 = local read "Focus Index"() -> (w2526:sgl)
        n619 = Not(x=w2455) -> (.not. x?=w2454:bool)
        n620 = Compound Arithmetic op=AND(w2401, w2454) -> (w2456:bool)
        n621 = Greater Or Equal?(x=w2526, y=w2529) -> (x >= y?=w2528:bool)
        n622 = case shown="True" w2456 {
          tunnel: "FI Detector" -> [_ w2814]
          tunnel: w2457 -> [_ w2813]
          frame False {
            n623 = call <vilib>:"Draw Rectangle.vi"("picture"=picture data[5B], "rect"=T46 {"left"=0, "top"=0, "right"=0, "bottom"=0}) -> ("new picture"=w2810:picture)  [unwired: 7 in]
            n624 = property on="Detector A" class="IntGraph (strict)"("PlotImages.Front"=w2810) -> ()  [unwired: 2 in, 2 out]
            n625 = property on="Detector B" class="IntGraph (strict)"("PlotImages.Front"=w2810) -> ()  [unwired: 2 in, 2 out]
            n626 = property on="Det A" class="IntGraph (strict)"("PlotImages.Front"=w2810) -> ()  [unwired: 2 in, 2 out]
            n627 = property on="Det B" class="IntGraph (strict)"("PlotImages.Front"=w2810) -> ()  [unwired: 2 in, 2 out]
          }
          frame True {
            n628 = stacked-sequence {
              tunnel: w2814 -> [w2834 w2850]
              tunnel: w2813 -> [w2829 _]
              frame #0 {
                n629 = local read "Focus Index Options"() -> (w2823:T28)
                n630 = shared-variable ".\\Zeiss Library.lvlib\\Completed tile index"() -> (w2818:u8[])  [unwired: 1 in, 1 out]
                n631 = local read "Image fit to"() -> (w2815:u8)
                n632 = shared-variable ".\\Zeiss Library.lvlib\\Y resolution"() -> (w2819:u32)  [unwired: 1 in, 1 out]
                n633 = shared-variable ".\\Zeiss Library.lvlib\\X resolution"() -> (w2820:u32)  [unwired: 1 in, 1 out]
